vi "FTW-Message-Request-Unknown.vi"(8 "error in":errorcluster, 11 "FTW Incoming Request":refnum<class "FTW-Message-IncomingRequest.lvclass">) -> (0 "error out":errorcluster)   [LabVIEW 2012, in "FTW-Actor.lvlib" / "FTW-Message-IncomingRequest.lvclass"]
uses:
  FTW-Message-IncomingRequest.lvclass
panel:
  # "Inputs"
  # "Outputs"
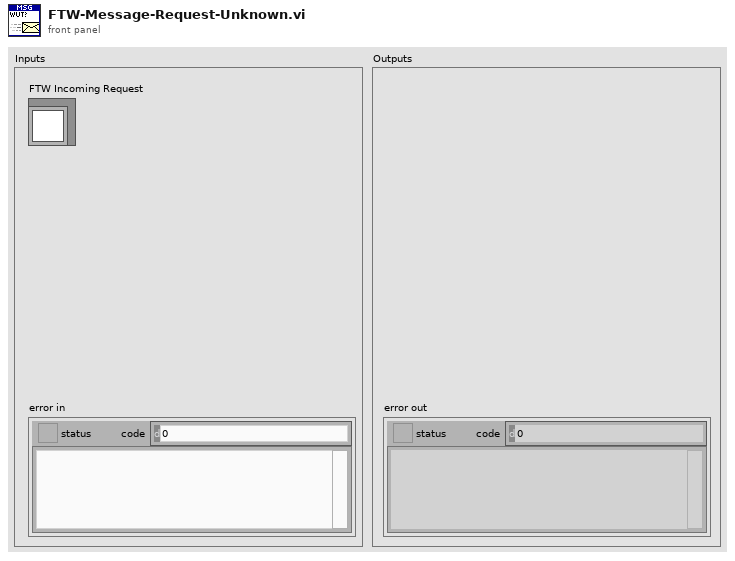
[diagram p1: front panel]
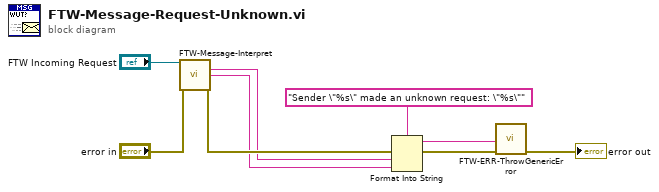
[diagram p0: block diagram]
diagram:
  n1 = call-dynamic "FTW-Message-Interpret.vi"("FTW Message"="FTW Incoming Request", "error in"="error in") -> ("Sender Identity"=w2:string, "Message Header"=w1:string, "error out"=w4:errorcluster)  [unwired: 9 in, 2 out]
  n2 = Format Into String(format string="Sender \"%s\" made an unknown request: \"%s\"", error in=w4, w2, w1) -> (resulting string=w5:string, error out=w6:errorcluster)  [unwired: 1 in]
  n3 = call "FTW-ERR-ThrowGenericError.vi"("Error Message"=w5, "error in"=w6) -> ("error out"=→"error out":errorcluster)  [unwired: 13 in]
